vi "Drive_Distance.vi"(1 "Timeout (ms)":dbl, 2 "Acceptable Error (in)":dbl, 3 "Distance (in)":dbl) -> (0 "Error (in)":dbl)   [LabVIEW 2020]
uses:
  <vilib>/Rock Robotics/WPI/ThirdParty/REV Robotics/REVLib/Typedef/Spark MAX Control Type.ctl
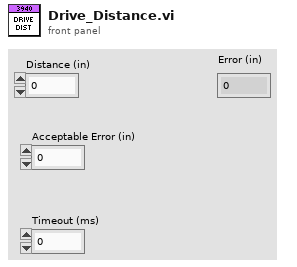
[diagram p1: front panel]
types:
  T1 = typedef "Spark MAX Control Type.ctl" = enum16{"Percent VBus", "Voltage", "Velocity", "Position", "Smart Motion", "Current", "Smart Velocity"}
  T2 = cluster{"P Gain":dbl, "I Gain":dbl, "D Gain":dbl, "F Gain":dbl, "I Zone":dbl, "Min Output":dbl, "Max Output":dbl}
  T3 = typedef "WPI_MotorControlDeviceRef.ctl" = cluster{"DeviceStatus":errorcluster, "Type":T4, "PWM":cluster{"PWM Channel":T5, "DeadBand":T6}, "CAN":cluster{"Device Number":u8, "SetOutput VI Ref":variant, "GetOutput VI Ref":variant, "Enable VI Ref":variant, "Disable VI Ref":variant, "Data":variant}, "Invert":bool, "DIO PWM":cluster{"PWM \"Enable\" Channel":T5, "DIOChannel":T7, "PWM Rate":dbl}}
  T4 = typedef "WPI_MotorControlType.ctl" = enum16{"PWM", "CAN", "DIO PWM"}
  T5 = typedef "FPGA_DIOPWMChannel.ctl" = enum8{"PWM 0", "PWM 1", "PWM 2", "PWM 3", "PWM 4", "PWM 5", "PWM 6", "PWM 7", "PWM 8", "PWM 9", "PWM MXP 0", "PWM MXP 1", "PWM MXP 2", "PWM MXP 3", "PWM MXP 4", "PWM MXP 5", "PWM MXP 6", "PWM MXP 7", "PWM MXP 8", "PWM MXP 9", "Invalid"}
  T6 = typedef "WPI_PWMDeadband.ctl" = cluster{"Name":string, "maxPositivePwm":i32, "minPositivePwm":i32, "centerPwm":i32, "maxNegativePwm":i32, "minNegativePwm":i32, "angularRange":u16}
  T7 = typedef "FPGA_DIOChannel.ctl" = enum8{"DIO 0", "DIO 1", "DIO 2", "DIO 3", "DIO 4", "DIO 5", "DIO 6", "DIO 7", "DIO 8", "DIO 9", "DIO MXP 0", "DIO MXP 1", "DIO MXP 2", "DIO MXP 3", "DIO MXP 4", "DIO MXP 5", "DIO MXP 6", "DIO MXP 7", "DIO MXP 8", "DIO MXP 9", "DIO MXP 10", "DIO MXP 11", "DIO MXP 12", "DIO MXP 13", "DIO MXP 14", "DIO MXP 15", "SPI Port CS1", "SPI Port CS2", "SPI Port CS3", "SPI Port MISO", "SPI Port MOSI", "Invalid"}
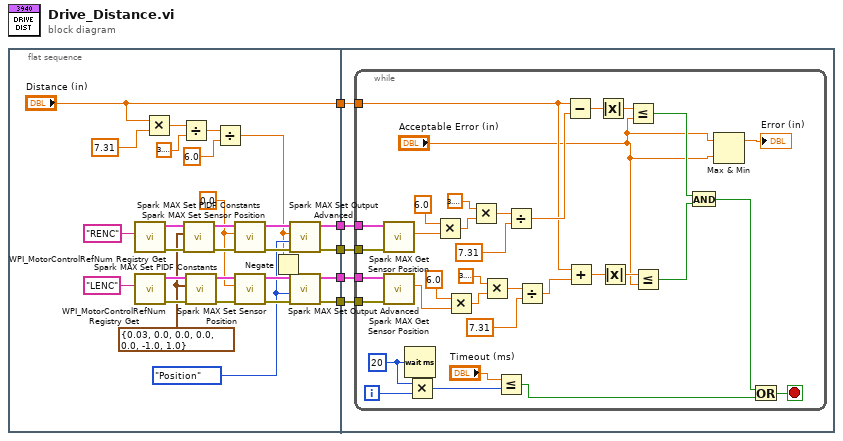
[diagram p0: block diagram]
diagram:
  n1 = flat-sequence {
    tunnel: [w11] -> w5
    tunnel: [w10] -> w4
    tunnel: [w9] -> w3
    tunnel: [w8] -> w2
    tunnel: ["Distance (in)"] -> w1
    tunnel: w5 -> [w39]
    tunnel: w4 -> [w38]
    tunnel: w3 -> [w37]
    tunnel: w2 -> [w36]
    tunnel: w1 -> [w35]
    frame #0 {
      w18 = Spark_MAX_Control_Type."Position" ("Control Mode")
      w19 = T2 {"P Gain"=0.03, "I Gain"=0.0, "D Gain"=0.0, "F Gain"=0.0, "I Zone"=0.0, "Min Output"=-1.0, "Max Output"=1.0} ("PID Constants")
      w20 = 0.0 ("Position")
      n2 = call <vilib>:"WPI_MotorControlRefNum Registry Get.vi"("refnum name"="RENC") -> ("error out"=w32:errorcluster, "MotorControlDevRef"=w31:T3)  [unwired: 9 in]
      n3 = call <vilib>:"WPI_MotorControlRefNum Registry Get.vi"("refnum name"="LENC") -> ("error out"=w30:errorcluster, "MotorControlDevRef"=w29:T3)  [unwired: 9 in]
      n4 = Multiply(x="Distance (in)", y=7.31) -> (x*y=w16:dbl)
      n5 = Divide(x=w16, y=3.141592653589793) -> (x/y=w14:dbl)
      n6 = call <vilib>:"Spark MAX Set PIDF Constants.vi"("error in"=w32, "PID Constants"=w19, "MotorControlDeviceRef"=w31) -> ("error out"=w28:errorcluster, "MotorControlDeviceRef"=w27:T3)  [unwired: 7 in]
      n7 = call <vilib>:"Spark MAX Set PIDF Constants.vi"("error in"=w30, "PID Constants"=w19, "MotorControlDeviceRef"=w29) -> ("error out"=w26:errorcluster, "MotorControlDeviceRef"=w25:T3)  [unwired: 7 in]
      n8 = Divide(x=w14, y=6.0) -> (x/y=w12:dbl)
      n9 = call <vilib>:"Spark MAX Set Sensor Position.vi"("error in"=w28, "Position"=w20, "MotorControlDeviceRef"=w27) -> ("error out"=w24:errorcluster, "MotorControlDeviceRef"=w23:T3)  [unwired: 7 in]
      n10 = call <vilib>:"Spark MAX Set Sensor Position.vi"("error in"=w26, "Position"=w20, "MotorControlDeviceRef"=w25) -> ("error out"=w22:errorcluster, "MotorControlDeviceRef"=w21:T3)  [unwired: 7 in]
      n11 = Negate(x=w12) -> (-x=w7:dbl)
      n12 = call <vilib>:"Spark MAX Set Output Advanced.vi"("error in (no error)"=w24, "Control Mode"=w18, "Setpoint"=w12, "MotorControlDevRef"=w23) -> ("error out"=w8:errorcluster, "MotorControlDevRef"=w11:T3)  [unwired: 6 in]
      n13 = call <vilib>:"Spark MAX Set Output Advanced.vi"("error in (no error)"=w22, "Control Mode"=w18, "Setpoint"=w7, "MotorControlDevRef"=w21) -> ("error out"=w9:errorcluster, "MotorControlDevRef"=w10:T3)  [unwired: 6 in]
    }
    frame #1 {
      n14 = while {
        tunnel: w39 -> [w73]
        tunnel: w38 -> [w72]
        tunnel: w37 -> [w71]
        tunnel: w36 -> [w70]
        tunnel: w35 -> [w53]
        i -> [w48]
        stop <- w42 stop-if-true
        w47 = u32 20 ("milliseconds to wait")
        n15 = call <vilib>:"Spark MAX Get Sensor Position.vi"("error in (no error)"=w70, "MotorControlDevRef in"=w73) -> ("Sensor Position"=w69:dbl)  [unwired: 6 in, 3 out]
        n16 = call <vilib>:"Spark MAX Get Sensor Position.vi"("error in (no error)"=w71, "MotorControlDevRef in"=w72) -> ("Sensor Position"=w55:dbl)  [unwired: 6 in, 3 out]
        n17 = Wait (ms)(milliseconds to wait=w47) -> ()  [unwired: 1 out]
        n18 = Multiply(x=w47, y=w48) -> (x*y=w46:u32)
        n19 = Multiply(x=6.0, y=w69) -> (x*y=w67:dbl)
        n20 = Multiply(x=6.0, y=w55) -> (x*y=w59:dbl)
        n21 = Multiply(x=3.141592653589793, y=w67) -> (x*y=w65:dbl)
        n22 = Multiply(x=3.141592653589793, y=w59) -> (x*y=w57:dbl)
        n23 = Less Or Equal?(x="Timeout (ms)", y=w46) -> (x <= y?=w44:bool)
        n24 = Divide(x=w65, y=7.31) -> (x/y=w63:dbl)
        n25 = Divide(x=w57, y=7.31) -> (x/y=w54:dbl)
        n26 = Subtract(x=w53, y=w63) -> (x-y=w62:dbl)
        n27 = Add(x=w53, y=w54) -> (x+y=w52:dbl)
        n28 = Absolute Value(x=w62) -> (abs(x)=w61:dbl)
        n29 = Absolute Value(x=w52) -> (abs(x)=w51:dbl)
        n30 = Less Or Equal?(x=w61, y="Acceptable Error (in)") -> (x <= y?=w50:bool)
        n31 = Less Or Equal?(x=w51, y="Acceptable Error (in)") -> (x <= y?=w49:bool)
        n32 = And(x=w50, y=w49) -> (x .and. y?=w43:bool)
        n33 = Max & Min(x="Acceptable Error (in)", y="Acceptable Error (in)") -> (max(x,y)=→"Error (in)":dbl)  [unwired: 1 out]
        n34 = Or(x=w43, y=w44) -> (x .or. y?=w42:bool)
      }
    }
  }
